vi "Refresh Flat BOM View.vi"(8 "Error in":errorcluster caption="Error in (no error)", 11 "Tree":refnum<vi>) -> (0 "Error out":errorcluster)   [LabVIEW 2018]
uses:
  TypeDef/Refresh Hierarchy View - States.ctl
  TypeDef/BOM Table Raw Items.ctl
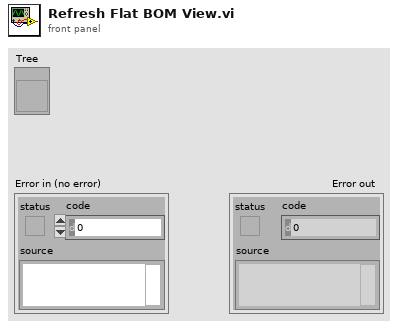
[diagram p1: front panel]
types:
  T1 = typedef "Refresh Hierarchy View - States.ctl" = enum16{"Defer Panel Updates", "Cleanup Tree", "Set Up Columns", "Set Up Rows", "Ping API", "GET BOM Rows", "Populate Table", "Adjust Column Width", "Release Panel Updates", "Exit"}
  T2 = typedef "BOM Table Raw Items.ctl" = cluster{"id":i32, "Full PN":string, "External Part Number":string, "Item description":string, "Part Number":string, "Revision":string, "Containing":cluster{"id":i32, "value":string}[], "Contained by":cluster{"id":i32, "value":string}[], "Part of a set":cluster{"id":i32}[]}
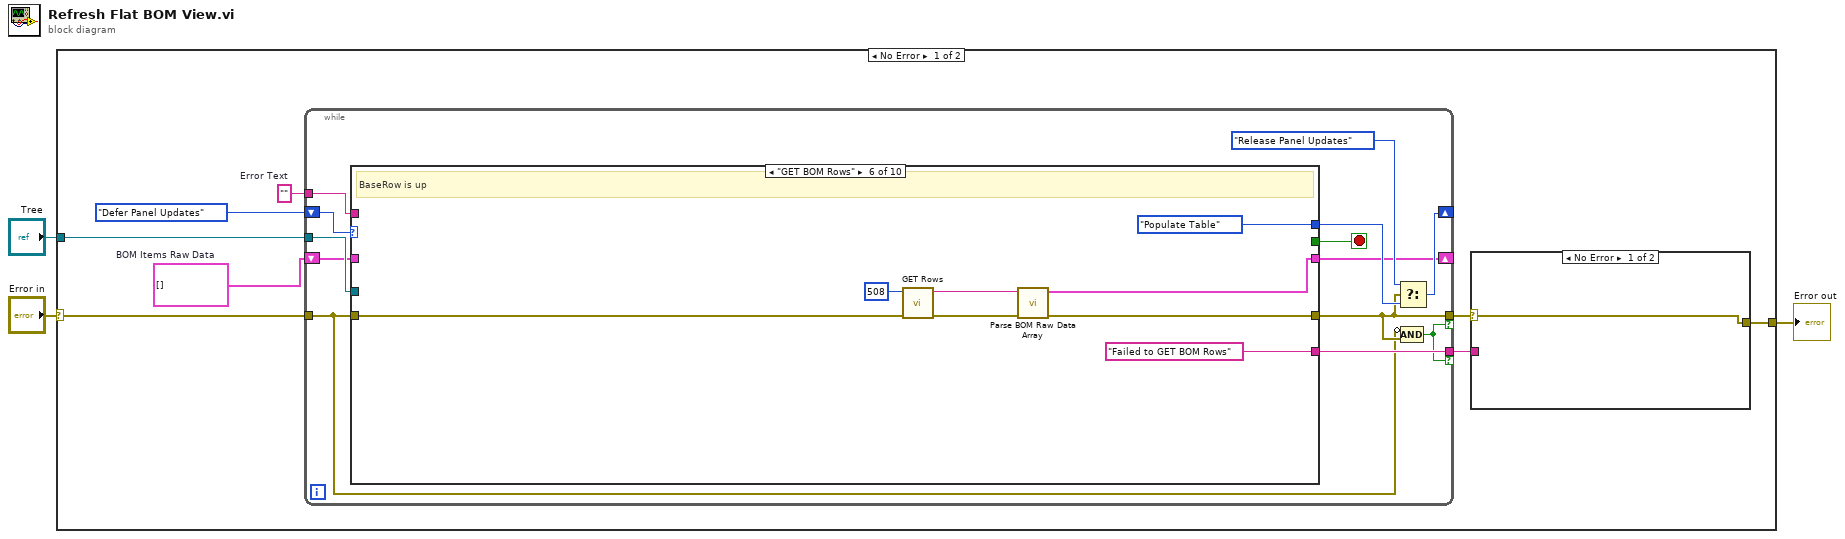
[diagram p0: block diagram]
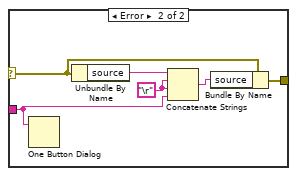
[diagram p2: hidden frame]
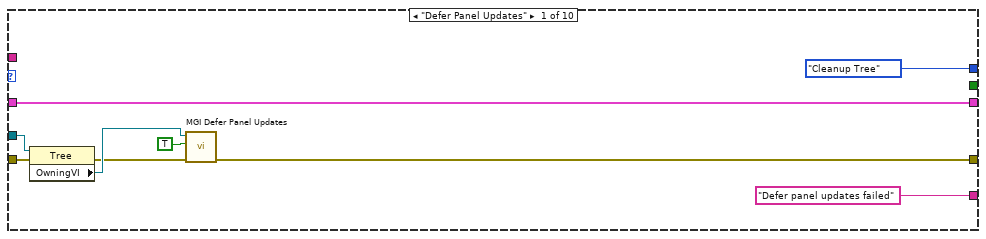
[diagram p3: hidden frame]
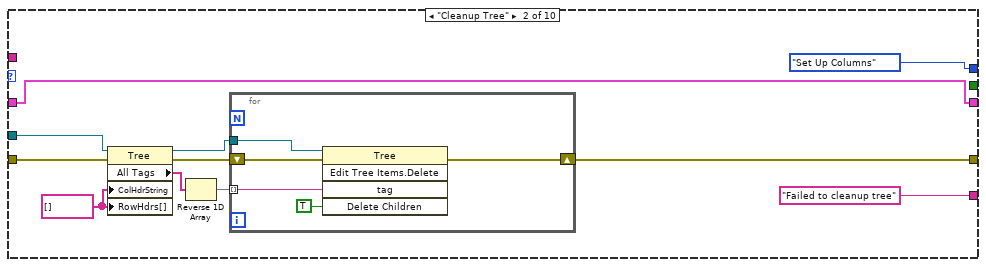
[diagram p4: hidden frame]
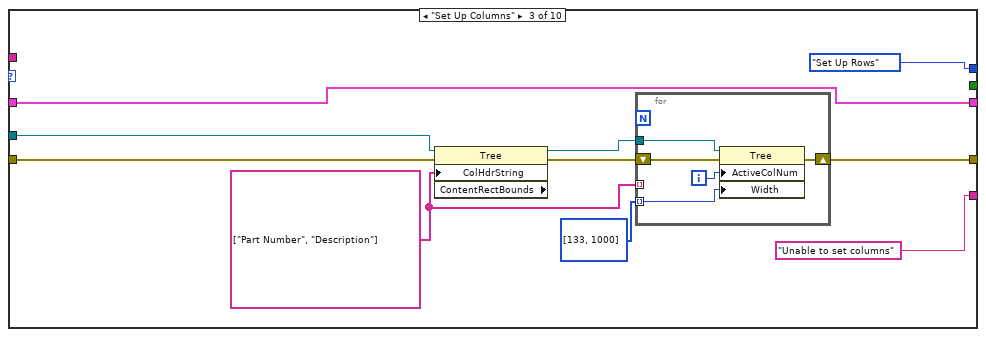
[diagram p5: hidden frame]
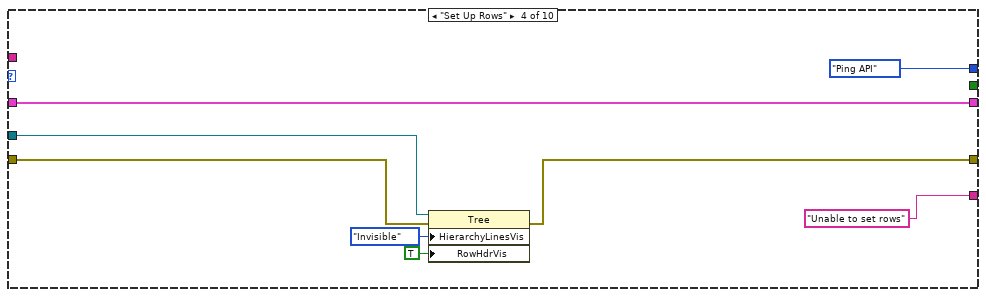
[diagram p6: hidden frame]
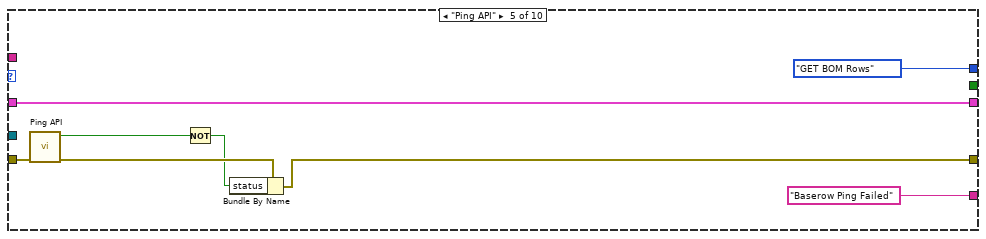
[diagram p7: hidden frame]
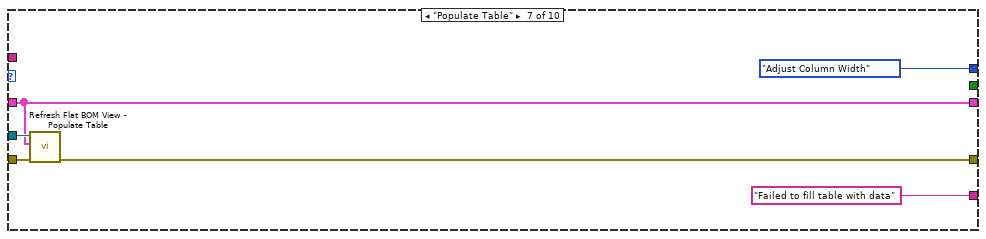
[diagram p8: hidden frame]
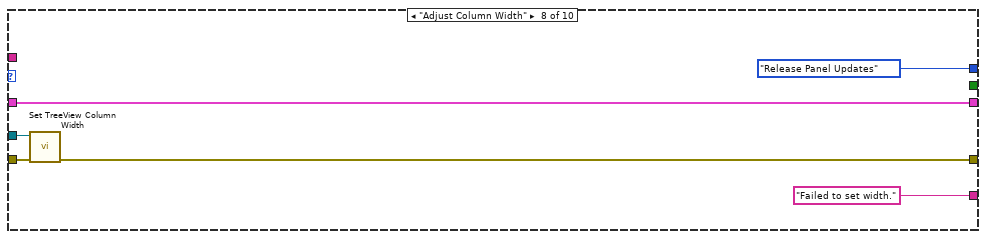
[diagram p9: hidden frame]
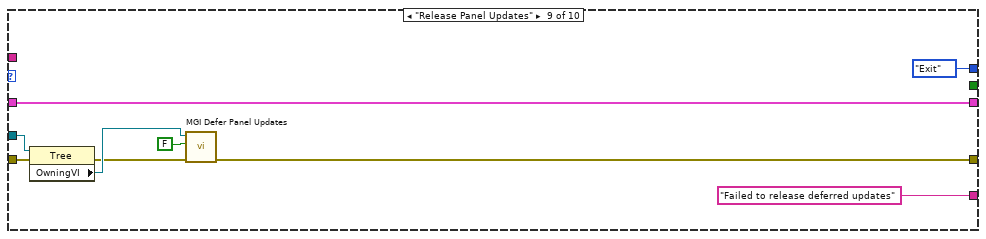
[diagram p10: hidden frame]
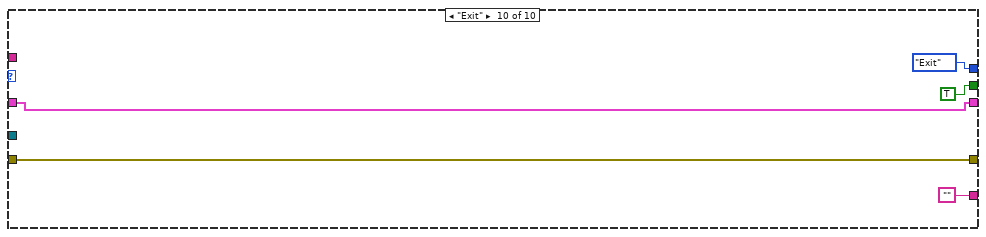
[diagram p11: hidden frame]
diagram:
  n1 = case shown="No Error" "Error in" {
    selector: "Error in" -> [w4 w122]
    tunnel: "Tree" -> [w9 _]
    tunnel: [w5 w122] -> w2
    frame No Error {
      w8 = T2[] []  # BOM Items Raw Data
      w10 = ""  # Error Text
      n2 = while {
        tunnel: w9 -> [w28]
        shift-right: [w26] -> _
        shift-left: Refresh_Hierarchy_View_-_States."Defer Panel Updates" -> [w31]
        shift-right: [w23] -> _
        shift-left: w8 -> [w22]
        tunnel: [w21] -> w7 if=w20
        tunnel: w10 -> [w29]
        tunnel: [w24] -> w6 if=w20
        tunnel: w4 -> [w19]
        stop <- w30 stop-if-true
        n3 = case shown="\"GET BOM Rows\"" w31 {
          tunnel: [w37 w45 w57 w75 w85 w91 w99 w103 w113 w120] -> w21
          tunnel: w19 -> [w35 w50 w65 w74 w87 w94 w98 w102 w111 w120]
          tunnel: [_ _ _ _ _ _ _ _ _ TRUE] -> w30
          tunnel: w29 -> [_ _ _ _ _ _ _ _ _ _]
          tunnel: w28 -> [w40 w51 w66 w76 _ _ w100 w104 w116 _]
          tunnel: [Refresh_Hierarchy_View_-_States."Cleanup Tree" Refresh_Hierarchy_View_-_States."Set Up Columns" Refresh_Hierarchy_View_-_States."Set Up Rows" Refresh_Hierarchy_View_-_States."Ping API" Refresh_Hierarchy_View_-_States."GET BOM Rows" Refresh_Hierarchy_View_-_States."Populate Table" Refresh_Hierarchy_View_-_States."Adjust Column Width" Refresh_Hierarchy_View_-_States."Release Panel Updates" Refresh_Hierarchy_View_-_States."Exit" Refresh_Hierarchy_View_-_States."Exit"] -> w27
          tunnel: ["Defer panel updates failed" "Failed to cleanup tree" "Unable to set columns" "Unable to set rows" "Baserow Ping Failed" "Failed to GET BOM Rows" "Failed to fill table with data" "Failed to set width." "Failed to release deferred updates" ""] -> w24
          tunnel: [w32 w41 w62 w79 w80 w88 w96 w107 w109 w117] -> w23
          tunnel: w22 -> [w32 w41 w62 w79 w80 _ w96 w107 w109 w117]
          frame "Defer Panel Updates" {
            n4 = property class="Tree"(reference=w40, error in=w35) -> (error out=w36:errorcluster, "OwningVI"=w39:refnum<vi>)  [unwired: 1 out]
            n5 = call <userlib>:"MGI Defer Panel Updates.vi"("Error In"=w36, "Defer Updates?"=TRUE, "VI Reference (Caller)"=w39) -> ("Error Out"=w37:errorcluster)  [unwired: 8 in]
          }
          frame "Cleanup Tree" {
            w44 = string[] [] ("Column Header Strings[]")
            n6 = property class="Tree"(reference=w51, error in=w50, "ColHdrString"=w44, "RowHdrs[]"=w44) -> (reference out=w48:refnum<vi>, error out=w46:errorcluster, "All Tags"=w49:string[])
            n7 = Reverse 1D Array(array=w49) -> (reversed array=w47:string[])
            n8 = for {
              tunnel: w48 -> [w56]
              tunnel: w47 -> [w55] mode=indexing
              shift-right: [w52] -> w45
              shift-left: w46 -> [w53]
              n9 = invoke class="Tree" method="Edit Tree Items.Delete"(reference=w56, error in=w53, "tag"=w55, "Delete Children"=TRUE ("Delete Children?")) -> (error out=w52:errorcluster)  [unwired: 1 in, 4 out]
            }
          }
          frame "Set Up Columns" {
            w61 = string[] ["Part Number", "Description"] ("Column Header Strings[]")
            n10 = property class="Tree" props=["ColHdrString", "ContentRectBounds"](reference=w66, error in=w65, "ColHdrString"=w61) -> (reference out=w59:refnum<vi>, error out=w58:errorcluster)  [unwired: 1 out]
            n11 = for {
              tunnel: w61 -> [_] mode=indexing
              tunnel: i32[] [133, 1000] ("Active Cell:Cell Size:Width") -> [w70] mode=indexing
              tunnel: w59 -> [w69]
              shift-right: [w67] -> w57
              shift-left: w58 -> [w68]
              i -> [w71]
              n12 = property class="Tree"(reference=w69, error in=w68, "ActiveColNum"=w71, "Width"=w70) -> (error out=w67:errorcluster)  [unwired: 1 out]
            }
          }
          frame "Set Up Rows" {
            n13 = property class="Tree"(reference=w76, error in=w74, "HierarchyLinesVis"=enum32{"Visible", "Invisible", "OS Default"}."Invisible" ("Visible Items:Hierarchy Lines Visible"), "RowHdrVis"=TRUE ("Visible Items:Row Headers Visible")) -> (error out=w75:errorcluster)  [unwired: 1 out]
          }
          frame "Ping API" {
            n14 = call "Ping API.vi"("Error in"=w87) -> ("Error out"=w86:errorcluster, "Connection OK"=w84:bool)  [unwired: 9 in]
            n15 = Not(x=w84) -> (.not. x?=w81:bool)
            n16 = Bundle By Name(cluster=w86, "status"=w81) -> (w85:errorcluster)
          }
          frame "GET BOM Rows" {
            # "BaseRow is up"
            n17 = call "GET Rows.vi"("Error in"=w94, "Table ID"=u32 508) -> ("Error out"=w92:errorcluster, "Rows Array JSON"=w93:string)  [unwired: 8 in]
            n18 = call "Parse BOM Raw Data Array.vi"("Error in"=w92, "BOM JSON String"=w93) -> ("Error out"=w91:errorcluster, "BOM Items Raw Data"=w88:T2[])  [unwired: 8 in]
          }
          frame "Populate Table" {
            n19 = call "Refresh Flat BOM View - Populate Table.vi"("error in (no error)"=w98, "BOM Items Raw Data"=w96, "TreeControl in"=w100) -> ("error out"=w99:errorcluster)  [unwired: 8 in]
          }
          frame "Adjust Column Width" {
            n20 = call "Set TreeView Column Width.vi"("error in (no error)"=w102, "TreeControl in"=w104) -> ("error out"=w103:errorcluster)  [unwired: 9 in]
          }
          frame "Release Panel Updates" {
            n21 = property class="Tree"(reference=w116, error in=w111) -> (error out=w112:errorcluster, "OwningVI"=w115:refnum<vi>)  [unwired: 1 out]
            n22 = call <userlib>:"MGI Defer Panel Updates.vi"("Error In"=w112, "Defer Updates?"=FALSE, "VI Reference (Caller)"=w115) -> ("Error Out"=w113:errorcluster)  [unwired: 8 in]
          }
          frame "Exit" {
          }
        }
        n23 = Select(t=Refresh_Hierarchy_View_-_States."Release Panel Updates", s=w21, f=w27) -> (s? t:f=w26:T1)
        n24 = Compound Arithmetic op=AND(invert w19, w21) -> (w20:bool)
      }
      n25 = case shown="No Error" w7 {
        selector: w7 -> [w12 w14]
        tunnel: w6 -> [_ w15]
        tunnel: [w12 w13] -> w5
        frame No Error {
        }
        frame Error {
          w17 = "\r"
          n26 = One Button Dialog(message=w15) -> ()  [unwired: 1 in, 1 out]
          n27 = Unbundle By Name(w14) -> ("source"=w18:string)
          n28 = Concatenate Strings(w18, w17, w17, w15) -> (w16:string)
          n29 = Bundle By Name(cluster=w14, "source"=w16) -> (w13:errorcluster)
        }
      }
    }
    frame Error {
    }
  }
  "Error out" <- w2
